vi "INTELLIFAUCET Stop.vi"(0 "Test Fixture Hardware":T2={"Power "={"Yokogawa"={"WT210"={"Sample Rate (1: 0.25s)"=1, "A Range (12: 20A)"=11, "V Range (6: 600V)"=4, "Power VISA Yokogawa WT210"="WT210"}, "WT500"={"Power VISA Yokogawa WT500"="", "V Range (8: 1000V)"=6, "I Range (7: 40A)"=7, "Update Rate (3: 500ms)"=2}, "WT310_2"={"Sample Rate (1: 0.25s)"=1, "A Range (12: 20A)"=11, "V Range (6: 600V)"=4, "Power VISA Yokogawa WT310_2"="WT310_2"}, "WT310_3"={"Sample Rate (1: 0.25s)"=1, "A Range (12: 20A)"=11, "V Range (6: 600V)"=4, "Power VISA Yokogawa WT310_3"="WT310_3"}}, "Aplus"={"Aplus IP Address"="192.168.1.101", "Remote Port"=502, "Instrument"="APLUS", "Instr Driver Revision"="1.03.0053"}, "Power Limits"={"Crest Factor"={"Upper Limit"=1.49, "Lower Limit"=1.34}, "Harmonic Content"={"Uthd"=2.0}, "Voltage"={"% Error"=2.0}, "Stability"={"<1 Watt "={"Wattage"=1.0, "Slope (mW/H)"=10.0}, ">1 Watt"={"1%Power/Hour"=1.0}}}, "Nominal Voltage"=120, "Time Limit (s)"=10800.0, "Power Variation Limit (%)"=50.0, "Power Supply"={"Chroma 61605"="CHROMA", "Use Chroma?"=FALSE}}, "Weight Scale"={"Com Options"={"IND560Scale VISA"="IND560", "IP Address"="", "Remote Port"=502, "Setra Scale VISA"="SETRA", "GSE 350"="GSE350"}, "Select Scale"=""}, "Flow Rates"={"Laurel Cold IP Address"="", "Laurel Hot IP Address"="", "Hot Water Laurel VISA"="LaurelMeter_Hot", "Cold Water Laurel VISA"="LaurelMeter_Cold", "Remote Port"=0, "Laurel Communication Type"="", "Meters To Collect (Hot Cold)"="", "HOT Laurel Reference"=refnum, "COLD Laurel Reference"=refnum, "Modbus Hot Ref"=refnum}, "Analog Data"={"Agilent"={"Agilent 34972_1"="34972A_1", "Agilent 34972_2"="34972A_2", "Agilent 34972_3"="34972A_3", "Agilent 34972_4"="34972A_3", "Agilent 34972_5"="34972A_3", "Agilent 34972_6"="34972A_3", "Agilent Gain"=0.0, "TC Type (K,J,T)"="", "Instrument IDN?"="", "TC Channels-List"="", "Analog Channels-List"="", "Agilent Cluster Array"=[], "TC Channels-List 2"="", "Analog Channels-List 2"=""}, "Yokogawa"={"MW100"="MW100", "Intellifaucet"=FALSE}, "Select Analog"="", "TC Coefficients"={"TC Coefficients 1"=[], "TC Coefficients 2"=[], "TC Coefficients 3"=[], "TC Coefficients 4"=[], "TC Coefficients 5"=[], "TC Coefficients 6"=[], "TC Coefficients 7"=[]}, "NI Tasks (Dryer DOE)"=["TC Temps-Module 1", "TC Temps-Module 2", "TC Temps-Module 3", "TC Temps-Module 4", "TC Temps-Module 5", "Gas and Temp-Module 6", "AC_DC Events-Module 7"], "Laurel Analog"={"Laurel IP (Water Temp)"="", "Laurel IP (Pressure)"=""}}, "Viasala Temperature & Humidity"={"IP Address 1"="", "Remote Port"=0, "IP Address 2"="", "IP Address 3"="", "Viasala Modbus"=refnum, "Probe Number"=0}, "Gas Meter"={"Gas Meter 1"="COM3", "Gas Meter 2"="COM4", "Gas Meter 3"="COM5", "Gas Meter 4"="COM6", "Gas Meter 5"="COM7", "Gas Meter 6"="COM8", "Data Frame Format"={"Absolute Pressure"=FALSE, "Gauge/Diff. Pressure"=FALSE, "Barometric Pressure"=FALSE, "Temperature"=FALSE, "Volumetric"=FALSE, "Mass"=FALSE, "Setpoint"=FALSE, "Valve Drive"=FALSE, "Totalizer"=FALSE, "Totalizer Timer"=FALSE, "Totalizer Average Flow"=FALSE, "Totalizer Peak Flow"=FALSE, "Gas Selected"=FALSE, "Tot. Timer Format"=0}, "Measurement Units"={"Software Rev"="", "Model Number"="", "Manufacturer Info"="", "Software Sub-Rev"="", "Board Rev"="", "Units of Measure Input"={"Abs. Pressure"="", "Gauge/Diff. Press."="", "Barometric Press."="", "Temperature"="", "Volume"="", "Mass"="", "Setpoint"="", "Valve Drive"="", "Totalizer"="", "Tot. Timer"="", "Tot. Avg. Flow"="", "Tot. Peak Flow"=""}}, "Ritter Gas Meter 1"="COM8"}, "Barometric Pressure"={"HEISE 901A"="HEISE", "Use Barometer?"=FALSE}, "Gas Analysis"={"Ultramat 23 VISA"="ULTRAMAT"}, "Inficon Micro GC"={"Propane IP Address"="192.168.1.33", "Natural Gas  IP Address"="192.168.1.32", "Remote Port"=502, "Natural Modbus"=refnum, "Propane Modbus"=refnum}, "Tenney Environmental Chamber"={"Remote Port"=0, "IP Address"="", "Tenney Modbus"=refnum}} {"Power"."Yokogawa"."WT310_3"."V Range (6: 600V)" items=["Auto", "15V", "30V", "60V", "150V", "300V", "600V"]; "Power"."Yokogawa"."WT310_3"."A Range (12: 20A)" items=["Auto", "5mA", "10mA", "20mA", "50mA", "100mA", "200mA", "0.5A", "1A", "2A", "5A", "10A", "20A", "50mV", "100mV", "200mV", "2.5V", "5V", "10V"]; "Power"."Yokogawa"."WT310_3"."Sample Rate (1: 0.25s)" items=["0.1s", "0.25s", "0.5s", "1s", "2s", "5s"]; "Power"."Yokogawa"."WT310_2"."V Range (6: 600V)" items=["Auto", "15V", "30V", "60V", "150V", "300V", "600V"]; "Power"."Yokogawa"."WT310_2"."A Range (12: 20A)" items=["Auto", "5mA", "10mA", "20mA", "50mA", "100mA", "200mA", "0.5A", "1A", "2A", "5A", "10A", "20A", "50mV", "100mV", "200mV", "2.5V", "5V", "10V"]; "Power"."Yokogawa"."WT310_2"."Sample Rate (1: 0.25s)" items=["0.1s", "0.25s", "0.5s", "1s", "2s", "5s"]; "Power"."Yokogawa"."WT500"."Update Rate (3: 500ms)" items=["-", "100ms", "200ms", "500ms", "1s", "2s", "5s"]; "Power"."Yokogawa"."WT500"."I Range (7: 40A)" items=["AUTO", "500 mA", "1 A", "2 A", "5 A", "10 A", "20 A", "40 A", "S-AUTO", "50 mV", "100 mV", "200 mV", "500 mV", "1 V", "2 V", "5 V", "10 V", "250 mA", "500 mA", "1 A", "2.5 A", "5 A", "10 A", "20 A", "25 mV", "50 mV", "100 mV", "250 mV", "500 mV", "1 V", "2.5 V", "5 V"]; "Power"."Yokogawa"."WT500"."V Range (8: 1000V)" items=["AUTO", "15", "30", "60", "100", "150", "300", "600", "1000", "7.5", "15", "30", "50", "75", "150", "300", "500"]; "Power"."Yokogawa"."WT210"."V Range (6: 600V)" items=["Auto", "15V", "30V", "60V", "150V", "300V", "600V"]; "Power"."Yokogawa"."WT210"."A Range (12: 20A)" items=["Auto", "5mA", "10mA", "20mA", "50mA", "100mA", "200mA", "0.5A", "1A", "2A", "5A", "10A", "20A", "50mV", "100mV", "200mV", "2.5V", "5V", "10V"]; "Power"."Yokogawa"."WT210"."Sample Rate (1: 0.25s)" items=["0.1s", "0.25s", "0.5s", "1s", "2s", "5s"]}, 1 "Mode":T1=enum."Stop Flow", 5 "mS wait":u32=200, 11 "Error In":errorcluster, 12 "Debug":bool, 13 "Refnum in":T12) -> (4 "Test Fixture Hardware Output":T2={"Power "={"Yokogawa"={"WT210"={"Sample Rate (1: 0.25s)"=1, "A Range (12: 20A)"=11, "V Range (6: 600V)"=4, "Power VISA Yokogawa WT210"="WT210"}, "WT500"={"Power VISA Yokogawa WT500"="", "V Range (8: 1000V)"=6, "I Range (7: 40A)"=7, "Update Rate (3: 500ms)"=2}, "WT310_2"={"Sample Rate (1: 0.25s)"=1, "A Range (12: 20A)"=11, "V Range (6: 600V)"=4, "Power VISA Yokogawa WT310_2"="WT310_2"}, "WT310_3"={"Sample Rate (1: 0.25s)"=1, "A Range (12: 20A)"=11, "V Range (6: 600V)"=4, "Power VISA Yokogawa WT310_3"="WT310_3"}}, "Aplus"={"Aplus IP Address"="192.168.1.101", "Remote Port"=502, "Instrument"="APLUS", "Instr Driver Revision"="1.03.0053"}, "Power Limits"={"Crest Factor"={"Upper Limit"=1.49, "Lower Limit"=1.34}, "Harmonic Content"={"Uthd"=2.0}, "Voltage"={"% Error"=2.0}, "Stability"={"<1 Watt "={"Wattage"=1.0, "Slope (mW/H)"=10.0}, ">1 Watt"={"1%Power/Hour"=1.0}}}, "Nominal Voltage"=120, "Time Limit (s)"=10800.0, "Power Variation Limit (%)"=50.0, "Power Supply"={"Chroma 61605"="CHROMA", "Use Chroma?"=FALSE}}, "Weight Scale"={"Com Options"={"IND560Scale VISA"="IND560", "IP Address"="", "Remote Port"=502, "Setra Scale VISA"="SETRA", "GSE 350"="GSE350"}, "Select Scale"=""}, "Flow Rates"={"Laurel Cold IP Address"="", "Laurel Hot IP Address"="", "Hot Water Laurel VISA"="LaurelMeter_Hot", "Cold Water Laurel VISA"="LaurelMeter_Cold", "Remote Port"=0, "Laurel Communication Type"="", "Meters To Collect (Hot Cold)"="", "HOT Laurel Reference"=refnum, "COLD Laurel Reference"=refnum, "Modbus Hot Ref"=refnum}, "Analog Data"={"Agilent"={"Agilent 34972_1"="34972A_1", "Agilent 34972_2"="34972A_2", "Agilent 34972_3"="34972A_3", "Agilent 34972_4"="34972A_3", "Agilent 34972_5"="34972A_3", "Agilent 34972_6"="34972A_3", "Agilent Gain"=0.0, "TC Type (K,J,T)"="", "Instrument IDN?"="", "TC Channels-List"="", "Analog Channels-List"="", "Agilent Cluster Array"=[], "TC Channels-List 2"="", "Analog Channels-List 2"=""}, "Yokogawa"={"MW100"="MW100", "Intellifaucet"=FALSE}, "Select Analog"="", "TC Coefficients"={"TC Coefficients 1"=[], "TC Coefficients 2"=[], "TC Coefficients 3"=[], "TC Coefficients 4"=[], "TC Coefficients 5"=[], "TC Coefficients 6"=[], "TC Coefficients 7"=[]}, "NI Tasks (Dryer DOE)"=["TC Temps-Module 1", "TC Temps-Module 2", "TC Temps-Module 3", "TC Temps-Module 4", "TC Temps-Module 5", "Gas and Temp-Module 6", "AC_DC Events-Module 7"], "Laurel Analog"={"Laurel IP (Water Temp)"="", "Laurel IP (Pressure)"=""}}, "Viasala Temperature & Humidity"={"IP Address 1"="", "Remote Port"=0, "IP Address 2"="", "IP Address 3"="", "Viasala Modbus"=refnum, "Probe Number"=0}, "Gas Meter"={"Gas Meter 1"="COM3", "Gas Meter 2"="COM4", "Gas Meter 3"="COM5", "Gas Meter 4"="COM6", "Gas Meter 5"="COM7", "Gas Meter 6"="COM8", "Data Frame Format"={"Absolute Pressure"=FALSE, "Gauge/Diff. Pressure"=FALSE, "Barometric Pressure"=FALSE, "Temperature"=FALSE, "Volumetric"=FALSE, "Mass"=FALSE, "Setpoint"=FALSE, "Valve Drive"=FALSE, "Totalizer"=FALSE, "Totalizer Timer"=FALSE, "Totalizer Average Flow"=FALSE, "Totalizer Peak Flow"=FALSE, "Gas Selected"=FALSE, "Tot. Timer Format"=0}, "Measurement Units"={"Software Rev"="", "Model Number"="", "Manufacturer Info"="", "Software Sub-Rev"="", "Board Rev"="", "Units of Measure Input"={"Abs. Pressure"="", "Gauge/Diff. Press."="", "Barometric Press."="", "Temperature"="", "Volume"="", "Mass"="", "Setpoint"="", "Valve Drive"="", "Totalizer"="", "Tot. Timer"="", "Tot. Avg. Flow"="", "Tot. Peak Flow"=""}}, "Ritter Gas Meter 1"="COM8"}, "Barometric Pressure"={"HEISE 901A"="HEISE", "Use Barometer?"=FALSE}, "Gas Analysis"={"Ultramat 23 VISA"="ULTRAMAT"}, "Inficon Micro GC"={"Propane IP Address"="192.168.1.33", "Natural Gas  IP Address"="192.168.1.32", "Remote Port"=502, "Natural Modbus"=refnum, "Propane Modbus"=refnum}, "Tenney Environmental Chamber"={"Remote Port"=0, "IP Address"="", "Tenney Modbus"=refnum}} {"Power"."Yokogawa"."WT310_3"."V Range (6: 600V)" items=["Auto", "15V", "30V", "60V", "150V", "300V", "600V"]; "Power"."Yokogawa"."WT310_3"."A Range (12: 20A)" items=["Auto", "5mA", "10mA", "20mA", "50mA", "100mA", "200mA", "0.5A", "1A", "2A", "5A", "10A", "20A", "50mV", "100mV", "200mV", "2.5V", "5V", "10V"]; "Power"."Yokogawa"."WT310_3"."Sample Rate (1: 0.25s)" items=["0.1s", "0.25s", "0.5s", "1s", "2s", "5s"]; "Power"."Yokogawa"."WT310_2"."V Range (6: 600V)" items=["Auto", "15V", "30V", "60V", "150V", "300V", "600V"]; "Power"."Yokogawa"."WT310_2"."A Range (12: 20A)" items=["Auto", "5mA", "10mA", "20mA", "50mA", "100mA", "200mA", "0.5A", "1A", "2A", "5A", "10A", "20A", "50mV", "100mV", "200mV", "2.5V", "5V", "10V"]; "Power"."Yokogawa"."WT310_2"."Sample Rate (1: 0.25s)" items=["0.1s", "0.25s", "0.5s", "1s", "2s", "5s"]; "Power"."Yokogawa"."WT500"."Update Rate (3: 500ms)" items=["-", "100ms", "200ms", "500ms", "1s", "2s", "5s"]; "Power"."Yokogawa"."WT500"."I Range (7: 40A)" items=["AUTO", "500 mA", "1 A", "2 A", "5 A", "10 A", "20 A", "40 A", "S-AUTO", "50 mV", "100 mV", "200 mV", "500 mV", "1 V", "2 V", "5 V", "10 V", "250 mA", "500 mA", "1 A", "2.5 A", "5 A", "10 A", "20 A", "25 mV", "50 mV", "100 mV", "250 mV", "500 mV", "1 V", "2.5 V", "5 V"]; "Power"."Yokogawa"."WT500"."V Range (8: 1000V)" items=["AUTO", "15", "30", "60", "100", "150", "300", "600", "1000", "7.5", "15", "30", "50", "75", "150", "300", "500"]; "Power"."Yokogawa"."WT210"."V Range (6: 600V)" items=["Auto", "15V", "30V", "60V", "150V", "300V", "600V"]; "Power"."Yokogawa"."WT210"."A Range (12: 20A)" items=["Auto", "5mA", "10mA", "20mA", "50mA", "100mA", "200mA", "0.5A", "1A", "2A", "5A", "10A", "20A", "50mV", "100mV", "200mV", "2.5V", "5V", "10V"]; "Power"."Yokogawa"."WT210"."Sample Rate (1: 0.25s)" items=["0.1s", "0.25s", "0.5s", "1s", "2s", "5s"]}, 15 "Error Out":errorcluster)   [LabVIEW 2023]
uses:
  MW100/Type Definitions/HEWH MW100 Channel Numbers.ctl
  Utility/Type Definitions/UTILITY Power Inputs Control.ctl
  Drivers/IND560 Scale Monitor/Type Definitions/IND560 Configuration.ctl
  Type Definitions/HEWH Agilent Cluster.ctl
  Utility/Type Definitions/UTILITY TC Coefficients.ctl
  Drivers/Alicat Gas Meter Driver/Sub-VIs/Data Frame.ctl
  Drivers/Alicat Gas Meter Driver/Sub-VIs/Units of Measure.ctl
  Drivers/Omega FMA-1600A Series Gas Flow Meter/Type Definitions/FMA1600A Units String.ctl
  Drivers/Omega FMA-1600A Series Gas Flow Meter/Type Definitions/FMA1600A COM Ports.ctl
  Washer DOE/Type Definitions/DOE Test Fixture Hardware.ctl
  Type Definitions/INTELLIFAUCET Set Mode.ctl
  <vilib>/NI/Modbus Library/API/Master/Modbus Master.lvclass
  Drivers/Inficon Fusion Micro GC/Type Definitions/Inficon IP Address.ctl
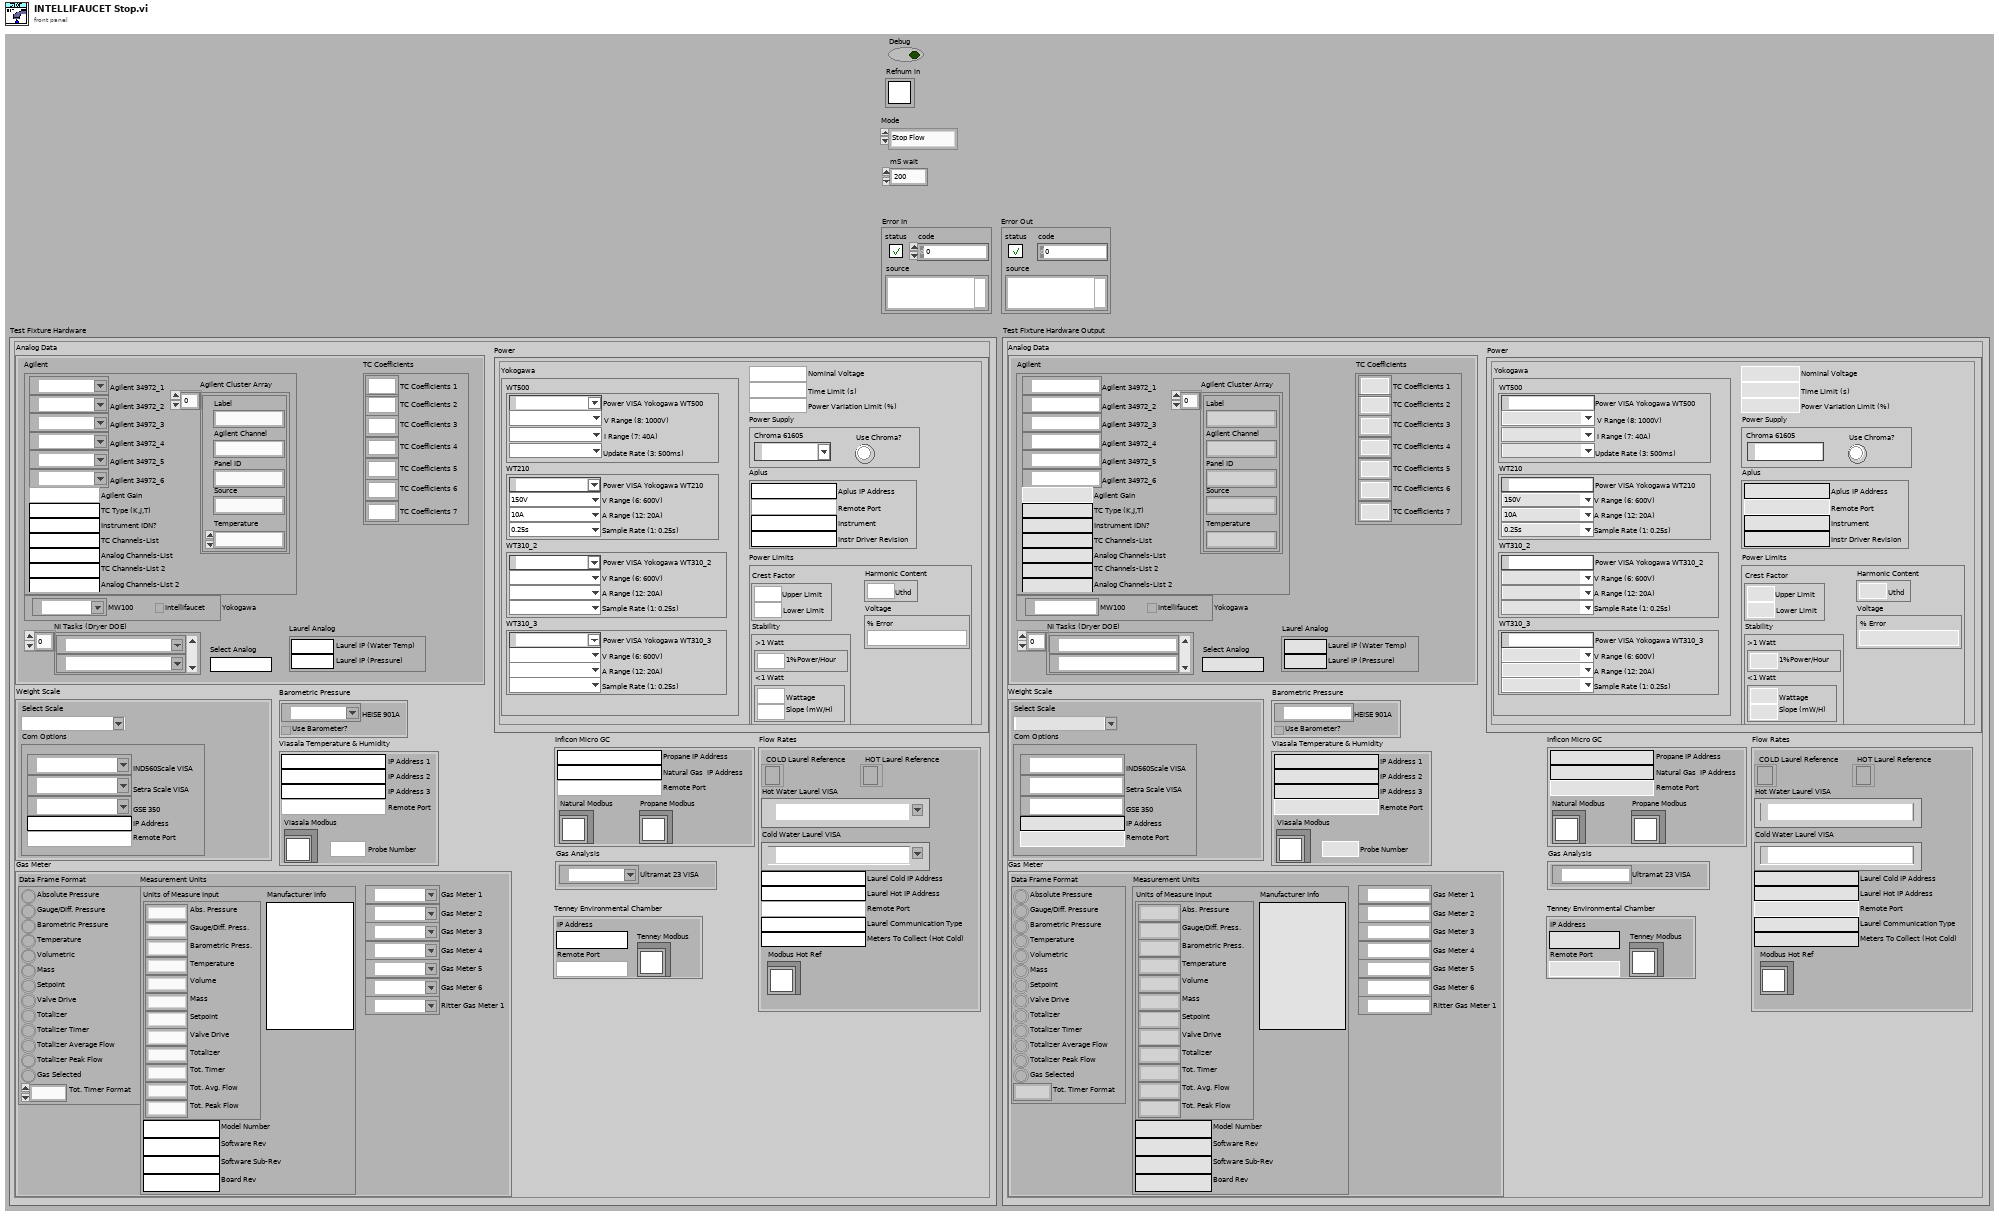
[diagram p1: front panel]
types:
  T1 = typedef "INTELLIFAUCET Set Mode.ctl" = enum16{"Adjust Temp", "Adjust Flow", "Start Flow", "Stop Flow", "Hold Start", "Hold Stop", "Release Start", "Release Stop", "Temp/Flow Relay", "Adjust Prop Valve"}
  T2 = typedef "DOE Test Fixture Hardware.ctl" = cluster{"Power ":T3, "Weight Scale":cluster{"Com Options":T4, "Select Scale":string}, "Flow Rates":cluster{"Laurel Cold IP Address":string, "Laurel Hot IP Address":string, "Hot Water Laurel VISA":refnum<visa-resource-name>, "Cold Water Laurel VISA":refnum<visa-resource-name>, "Remote Port":u16, "Laurel Communication Type":string, "Meters To Collect (Hot Cold)":string, "HOT Laurel Reference":refnum<k5>, "COLD Laurel Reference":refnum<k5>, "Modbus Hot Ref":refnum<class "Modbus Master.lvclass">}, "Analog Data":cluster{"Agilent":cluster{"Agilent 34972_1":refnum<visa-resource-name>, "Agilent 34972_2":refnum<visa-resource-name>, "Agilent 34972_3":refnum<visa-resource-name>, "Agilent 34972_4":refnum<visa-resource-name>, "Agilent 34972_5":refnum<visa-resource-name>, "Agilent 34972_6":refnum<visa-resource-name>, "Agilent Gain":dbl, "TC Type (K,J,T)":string, "Instrument IDN?":string, "TC Channels-List":string, "Analog Channels-List":string, "Agilent Cluster Array":T5[], "TC Channels-List 2":string, "Analog Channels-List 2":string}, "Yokogawa":cluster{"MW100":refnum<visa-resource-name>, "Intellifaucet":bool}, "Select Analog":string, "TC Coefficients":T6, "NI Tasks (Dryer DOE)":refnum<k21>[], "Laurel Analog":cluster{"Laurel IP (Water Temp)":string, "Laurel IP (Pressure)":string}}, "Viasala Temperature & Humidity":cluster{"IP Address 1":string, "Remote Port":u16, "IP Address 2":string, "IP Address 3":string, "Viasala Modbus":refnum<class "Modbus Master.lvclass">, "Probe Number":u16}, "Gas Meter":T7, "Barometric Pressure":cluster{"HEISE 901A":refnum<visa-resource-name>, "Use Barometer?":bool}, "Gas Analysis":cluster{"Ultramat 23 VISA":refnum<visa-resource-name>}, "Inficon Micro GC":T11, "Tenney Environmental Chamber":cluster{"Remote Port":u16, "IP Address":string, "Tenney Modbus":refnum<class "Modbus Master.lvclass">}}
  T3 = typedef "UTILITY Power Inputs Control.ctl" = cluster{"Yokogawa":cluster{"WT210":cluster{"Sample Rate (1: 0.25s)":i32, "A Range (12: 20A)":i32, "V Range (6: 600V)":i32, "Power VISA Yokogawa WT210":refnum<visa-resource-name>}, "WT500":cluster{"Power VISA Yokogawa WT500":refnum<visa-resource-name>, "V Range (8: 1000V)":i32, "I Range (7: 40A)":i32, "Update Rate (3: 500ms)":i32}, "WT310_2":cluster{"Sample Rate (1: 0.25s)":i32, "A Range (12: 20A)":i32, "V Range (6: 600V)":i32, "Power VISA Yokogawa WT310_2":refnum<visa-resource-name>}, "WT310_3":cluster{"Sample Rate (1: 0.25s)":i32, "A Range (12: 20A)":i32, "V Range (6: 600V)":i32, "Power VISA Yokogawa WT310_3":refnum<visa-resource-name>}}, "Aplus":cluster{"Aplus IP Address":string, "Remote Port":i32, "Instrument":string, "Instr Driver Revision":string}, "Power Limits":cluster{"Crest Factor":cluster{"Upper Limit":dbl, "Lower Limit":dbl}, "Harmonic Content":cluster{"Uthd":dbl}, "Voltage":cluster{"% Error":dbl}, "Stability":cluster{"<1 Watt ":cluster{"Wattage":dbl, "Slope (mW/H)":dbl}, ">1 Watt":cluster{"1%Power/Hour":dbl}}}, "Nominal Voltage":i32, "Time Limit (s)":dbl, "Power Variation Limit (%)":dbl, "Power Supply":cluster{"Chroma 61605":refnum<visa-resource-name>, "Use Chroma?":bool}}
  T4 = typedef "IND560 Configuration.ctl" = cluster{"IND560Scale VISA":refnum<visa-resource-name>, "IP Address":string, "Remote Port":u16, "Setra Scale VISA":refnum<visa-resource-name>, "GSE 350":refnum<visa-resource-name>}
  T5 = typedef "HEWH Agilent Cluster.ctl" = cluster{"Label":string, "Agilent Channel":string, "Panel ID":string, "Source":string, "Temperature":dbl}
  T6 = typedef "UTILITY TC Coefficients.ctl" = cluster{"TC Coefficients 1":dbl[], "TC Coefficients 2":dbl[], "TC Coefficients 3":dbl[], "TC Coefficients 4":dbl[], "TC Coefficients 5":dbl[], "TC Coefficients 6":dbl[], "TC Coefficients 7":dbl[]}
  T7 = typedef "FMA1600A COM Ports.ctl" = cluster{"Gas Meter 1":refnum<visa-resource-name>, "Gas Meter 2":refnum<visa-resource-name>, "Gas Meter 3":refnum<visa-resource-name>, "Gas Meter 4":refnum<visa-resource-name>, "Gas Meter 5":refnum<visa-resource-name>, "Gas Meter 6":refnum<visa-resource-name>, "Data Frame Format":T8, "Measurement Units":T9, "Ritter Gas Meter 1":refnum<visa-resource-name>}
  T8 = typedef "Data Frame.ctl" = cluster{"Absolute Pressure":bool, "Gauge/Diff. Pressure":bool, "Barometric Pressure":bool, "Temperature":bool, "Volumetric":bool, "Mass":bool, "Setpoint":bool, "Valve Drive":bool, "Totalizer":bool, "Totalizer Timer":bool, "Totalizer Average Flow":bool, "Totalizer Peak Flow":bool, "Gas Selected":bool, "Tot. Timer Format":u16}
  T9 = typedef "FMA1600A Units String.ctl" = cluster{"Software Rev":string, "Model Number":string, "Manufacturer Info":string, "Software Sub-Rev":string, "Board Rev":string, "Units of Measure Input":T10}
  T10 = typedef "Units of Measure.ctl" = cluster{"Abs. Pressure":string, "Gauge/Diff. Press.":string, "Barometric Press.":string, "Temperature":string, "Volume":string, "Mass":string, "Setpoint":string, "Valve Drive":string, "Totalizer":string, "Tot. Timer":string, "Tot. Avg. Flow":string, "Tot. Peak Flow":string}
  T11 = typedef "Inficon IP Address.ctl" = cluster{"Propane IP Address":string, "Natural Gas  IP Address":string, "Remote Port":u16, "Natural Modbus":refnum<class "Modbus Master.lvclass">, "Propane Modbus":refnum<class "Modbus Master.lvclass">}
  T12 = typedef "Semaphore RefNum" = refnum<k1>
  T13 = typedef "HEWH MW100 Channel Numbers.ctl" = string
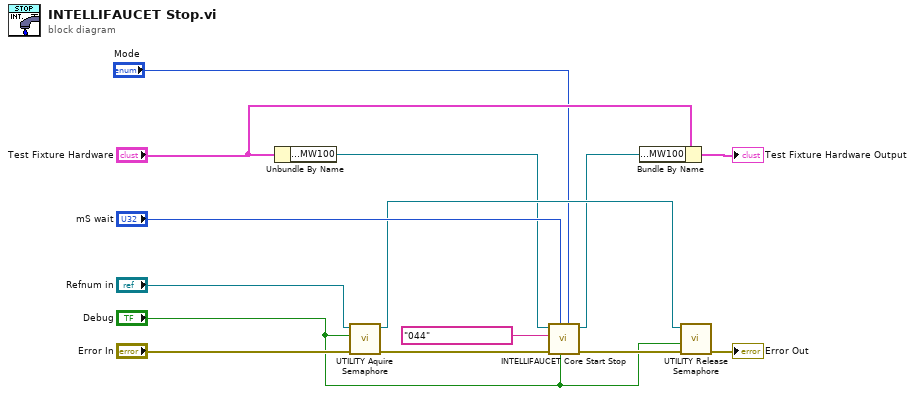
[diagram p0: block diagram]
diagram:
  n1 = Unbundle By Name("Test Fixture Hardware") -> ("Analog Data.Yokogawa.MW100"=w4:refnum<visa-resource-name>)
  n2 = call "UTILITY Aquire Semaphore.vi"("error in (no error)"="Error In", "Debug"="Debug", "Refnum in"="Refnum in") -> ("error out"=w9:errorcluster, "Refnum out"=w8:T12)  [unwired: 7 in]
  n3 = call "INTELLIFAUCET Core Start Stop.vi"("Mode"="Mode", "Debug"="Debug", "mS wait"="mS wait", "error in (no error)"=w9, "HEWH MW100 Channel Numbers"=T13 "044", "VISA Refnum in"=w4) -> ("error out"=w12:errorcluster, "VISA Refnum out"=w3:refnum<visa-resource-name>)  [unwired: 4 in]
  n4 = Bundle By Name(cluster="Test Fixture Hardware", "Analog Data.Yokogawa.MW100"=w3) -> (→"Test Fixture Hardware Output":T2)
  n5 = call "UTILITY Release Semaphore.vi"("error in (no error)"=w12, "Debug"="Debug", "Refnum in"=w8) -> ("error out"=→"Error Out":errorcluster)  [unwired: 8 in]
